vi "CreateSequenceLoop.vi"(10 "Active slaves":T2, 11 "scan control array":T3) -> (0 "Nscans":i32, 1 "Table 2":string[][](table) caption="Loop variable", 2 "output array":dbl[][](array[numeric]), 3 "scan header array":cluster{"Enum":T1, "variable name":string}[](array[cluster]), 4 "header":string[](array[string]))   [LabVIEW 2018, in "MasterProgramSupportFunctions.lvlib"]
uses:
  MasterProgramSupportFunctions.lvlib
  TargetScanControlArray.ctl
  VI_tags.ctl
  ActionSlaveVariable.ctl
  ActiveSlaves.ctl
  General Libraries/Sequences.lvlib
  MasterStatus.ctl
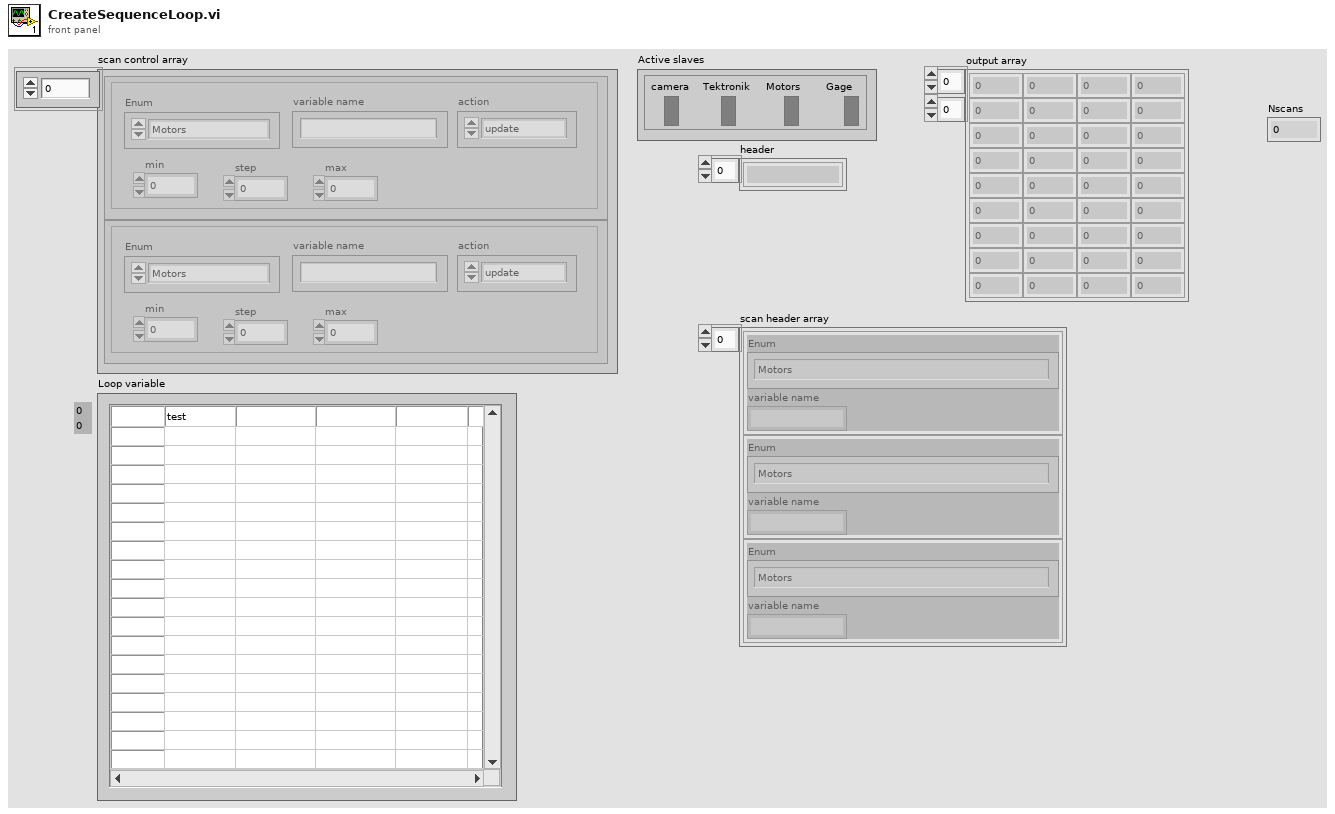
[diagram p1: front panel]
types:
  T1 = typedef "MasterProgramSupportFunctions.lvlib/VI_tags.ctl" = enum16{"Motors", "Gage", "Tektro3107", "XimeaMainCamera", "ContinuousMainScan"}
  T2 = typedef "MasterProgramSupportFunctions.lvlib/ActiveSlaves.ctl" = cluster{"camera":bool, "Tektronik":bool, "Motors":bool, "Gage":bool}
  T3 = typedef "MasterProgramSupportFunctions.lvlib/TargetScanControlArray.ctl" = cluster{"min":dbl, "step":dbl, "max":dbl, "Enum":T1, "variable name":string, "action":T4}[]
  T4 = typedef "MasterProgramSupportFunctions.lvlib/ActionSlaveVariable.ctl" = enum16{"update", "event"}
  T5 = cluster{"Camera done":bool, "Tektronik done":bool, "Motors done":bool, "Motors done 2":bool}
  T6 = cluster{"Camera done":bool, "Tektronik done":bool, "Motors done":bool, "Motors done 2":bool}[]
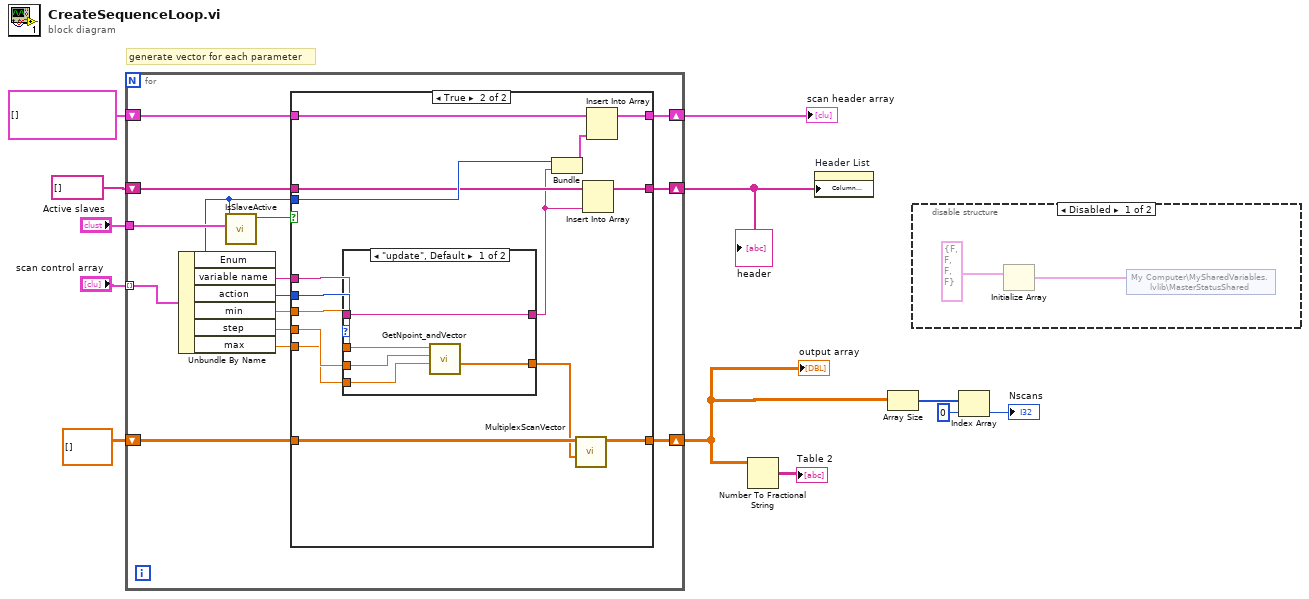
[diagram p0: block diagram]
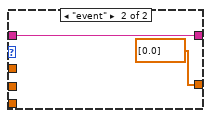
[diagram p4: hidden frame]
diagram:
  # "generate vector for each parameter"
  n1 = for {
    tunnel: "scan control array" -> [w27] mode=indexing
    tunnel: "Active slaves" -> [w26]
    shift-right: [w18] -> w4
    shift-left: dbl[][] [] ("output array") -> [w19]
    shift-right: [w17] -> w5
    shift-left: string[] [] -> [w16]
    shift-right: [w14] -> w6
    shift-left: cluster{"Enum":T1, "variable name":string}[] [] -> [w13]
    n2 = Unbundle By Name(w27) -> ("Enum"=w15:T1, "variable name"=w23:string, "action"=w24:T4, "min"=w22:dbl, "step"=w21:dbl, "max"=w20:dbl)
    n3 = call "IsSlaveActive.vi"("Active slaves"=w26, "Enum"=w15) -> ("camera"=w25:bool)  [unwired: 9 in]
    n4 = case shown="True" w25 {
      tunnel: w24 -> [_ w45]
      tunnel: w23 -> [_ w44]
      tunnel: w22 -> [_ w43]
      tunnel: w21 -> [_ w42]
      tunnel: w20 -> [_ w41]
      tunnel: w19 -> [w30 w40]
      tunnel: [w30 w38] -> w18
      tunnel: [w29 w37] -> w17
      tunnel: w16 -> [w29 w35]
      tunnel: w15 -> [_ w36]
      tunnel: [w28 w33] -> w14
      tunnel: w13 -> [w28 w31]
      frame False {
      }
      frame True {
        n5 = case shown="\"update\", Default" w45 {
          tunnel: w44 -> [w46 w51]
          tunnel: w43 -> [w50 _]
          tunnel: w42 -> [w49 _]
          tunnel: w41 -> [w48 _]
          tunnel: [w47 dbl[] [0.0] ("Point Array")] -> w39
          tunnel: [w46 w51] -> w32
          frame "update", Default {
            n6 = call "GetNpoint_andVector.vi"("max"=w48, "step"=w49, "min"=w50) -> ("Point Array"=w47:dbl[])  [unwired: 7 in, 1 out]
          }
          frame "event" {
          }
        }
        n7 = Bundle("Enum"=w36, "variable name"=w32) -> (w34:cluster{"Enum":T1, "variable name":string})  [unwired: 1 in]
        n8 = call "MultiplexScanVector.vi"("multiplyer"=w39, "initial matrix"=w40) -> ("output array"=w38:dbl[][])  [unwired: 9 in]
        n9 = Insert Into Array(array=w35, new element=w32) -> (w37:string[])  [unwired: 1 in]
        n10 = Insert Into Array(array=w31, new element=w34) -> (w33:cluster{"Enum":T1, "variable name":string}[])  [unwired: 1 in]
      }
    }
  }
  "output array" <- w4
  "scan header array" <- w6
  "header" <- w5
  n11 = Number To Fractional String(number=w4) -> (F-format string=→"Table 2":string[][])  [unwired: 3 in]
  n12 = property on="Header List" class="Tbl (strict)"("Column Headers[]"=w5) -> ()  [unwired: 2 in, 2 out]
  n13 = Array Size(array=w4) -> (size(s)=w3:i32[])
  n14 = disable-structure shown="Disabled" {
    frame Disabled {
      n15 = Initialize Array(T5 {"Camera done"=FALSE, "Tektronik done"=FALSE, "Motors done"=FALSE, "Motors done 2"=FALSE} ("Loop status bar")) -> (w53:T6)  [unwired: 1 in]
      n16 = shared-variable "My Computer\\MySharedVariables.lvlib\\MasterStatusShared"(w53) -> ()  [unwired: 1 in, 1 out]
    }
    frame Enabled {
    }
  }
  n17 = Index Array(array=w3, index=0) -> (element=→"Nscans":i32)
